vi "FpgaInterface.OpenFpga.vi"(8 "error in (no error)":errorcluster, 9 "Bitfile path":path, 10 "Device address":string="RIO0", 11 "PrivateData in":refnum<class "PrivateData.lvclass">) -> (0 "error out":errorcluster, 3 "PrivateData out":refnum<class "PrivateData.lvclass">)   [LabVIEW 2018, in "PrivateData.lvclass"]
uses:
  PrivateData.lvclass
  PrivateData.lvclass/PrivateData.ctl
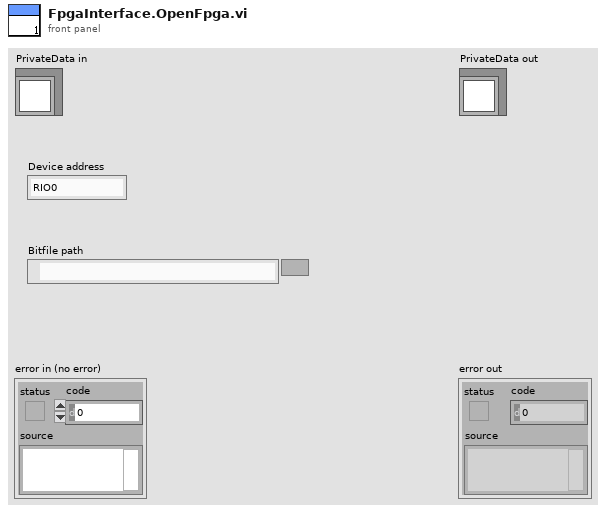
[diagram p1: front panel]
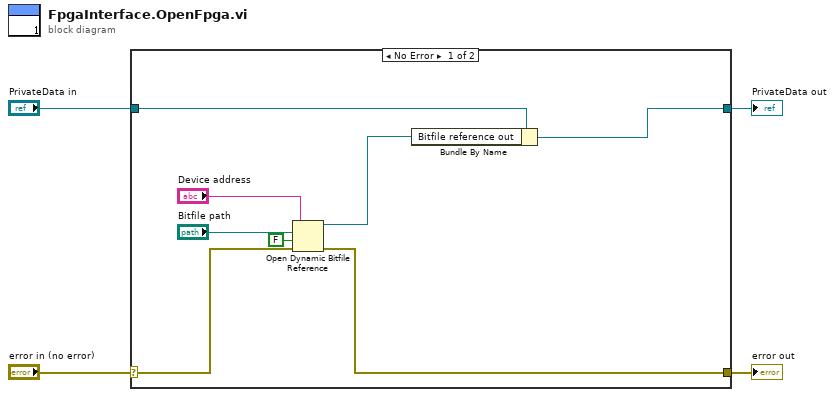
[diagram p0: block diagram]
diagram:
  n1 = case shown="No Error" "error in (no error)" {
    selector: "error in (no error)" -> [w11 w14]
    tunnel: [w8 w14] -> w3
    tunnel: [w5 w13] -> w1
    tunnel: "PrivateData in" -> [w7 w13]
    frame No Error {
      n2 = Open Dynamic Bitfile Reference(0:"Device address", 1:"Bitfile path", 2:FALSE ("Run When Loaded"), 3:w11) -> (5:w6:refnum<k20>, 8:w8:errorcluster)  [unwired: 1 in]
      n3 = Bundle By Name(cluster=w7, "Bitfile reference out"=w6) -> (w5:refnum<class "PrivateData.lvclass">)
    }
    frame Error {
    }
  }
  "error out" <- w3
  "PrivateData out" <- w1
